vi "SaveSC.vi"(8 "entrée d'erreur (pas d'erreur)":errorcluster, 11 "Control-Client en entrée":refnum<class "Control-Client.lvclass">) -> (0 "sortie d'erreur":errorcluster, 3 "Control-Client en sortie":refnum<class "Control-Client.lvclass">)   [LabVIEW 2020, in "Control-Client.lvclass"]
uses:
  Control-Client.lvclass
  Control-Client.lvclass/Control-Client.ctl
  methods/Read Group #.vi
  Experiments/Experiments_group.lvclass
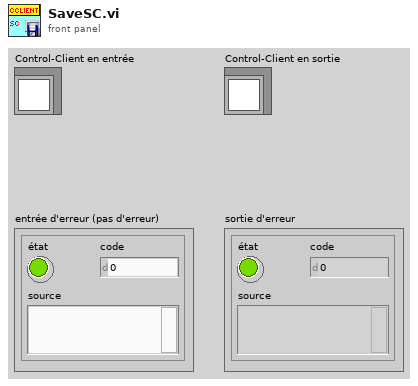
[diagram p1: front panel]
types:
  T1 = typedef "graphs_TR.ctl" = cluster{"TR SC":refnum<vi>, "TR OD":refnum<vi>, "Raw data":refnum<vi>, "Raw data BG":refnum<vi>}
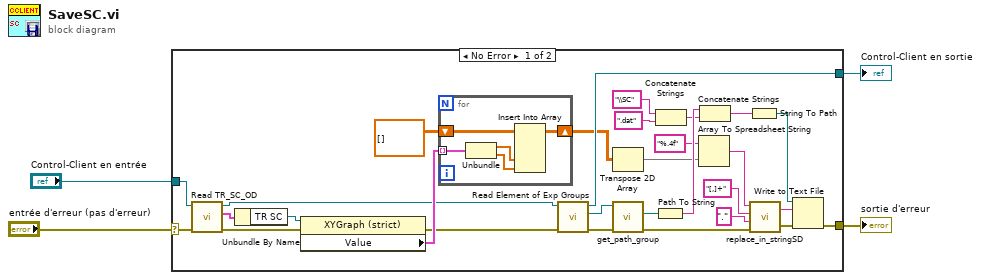
[diagram p0: block diagram]
diagram:
  n1 = case shown="No Error" "entrée d'erreur (pas d'erreur)" {
    selector: "entrée d'erreur (pas d'erreur)" -> [w11 w40]
    tunnel: [w33 w39] -> w4
    tunnel: [w32 w40] -> w3
    tunnel: "Control-Client en entrée" -> [w10 w39]
    frame No Error {
      n2 = call "Read TR_SC_OD.vi"("error in (no error)"=w11, "Control-Client en entrée"=w10) -> ("error out"=w7:errorcluster, "TR_SC_OD"=w9:T1, "Control-Client en sortie"=w5:refnum<class "Control-Client.lvclass">)  [unwired: 7 in]
      n3 = Unbundle By Name(w9) -> ("TR SC"=w8:refnum<vi>)
      n4 = property class="XYGraph (strict)"(reference=w8, error in=w7) -> (error out=w6:errorcluster, "Value"=w23:cluster{dbl[], dbl[]}[])  [unwired: 1 out]
      n5 = for {
        tunnel: w23 -> [w38] mode=indexing
        shift-right: [w34] -> w18
        shift-left: dbl[][] [] ("Tableau") -> [w37]
        n6 = Unbundle(w38) -> (w36:dbl[], w35:dbl[])
        n7 = Insert Into Array(array=w37, new element #1=w36, new element #2=w35) -> (w34:dbl[][])  [unwired: 2 in]
      }
      n8 = call "Read Element of Exp Groups.vi"("error in (no error)"=w6, "Control-Client in"=w5) -> ("error out"=w31:errorcluster, "Experiments_group.lvclass"=w13:refnum<class "Experiments_group.lvclass">, "Control-Client out"=w33:refnum<class "Control-Client.lvclass">)  [unwired: 7 in]
      n9 = Transpose 2D Array(2D array=w18) -> (transposed array=w19:dbl[][])
      n10 = call "get_path_group.vi"("error in (no error)"=w31, "Experiments_group.lvclass in"=w13) -> ("error out"=w14:errorcluster, "Path"=w26:path)  [unwired: 7 in, 1 out]
      n11 = Path To String(path=w26) -> (string=w29:string)
      n12 = Concatenate Strings("\\SC" ("chaîne"), ".dat" ("string")) -> (w28:string)
      n13 = Array To Spreadsheet String(array=w19, 3:"%.4f" ("chaîne de format")) -> (spreadsheet string=w22:string)  [unwired: 1 in]
      n14 = Concatenate Strings(w29, w28) -> (w27:string)
      n15 = String To Path(string=w27) -> (path=w24:path)
      n16 = call "replace_in_stringSD.vi"("error in (no error)"=w14, "replaced to.."=".", "characters to replace"="[,]+", "input string"=w22) -> ("error out"=w16:errorcluster, "output string"=w17:string)
      n17 = Write to Text File(file (use dialog)=w24, text=w17, error in=w16) -> (error out=w32:errorcluster)  [unwired: 1 in, 2 out]
    }
    frame Error {
    }
  }
  "Control-Client en sortie" <- w4
  "sortie d'erreur" <- w3
